vi "GetWaveformData.vi"(5 "Waveform Length (sec)":dbl, 7 "Number of Samples":i32, 8 "error in (no error)":errorcluster, 10 "Waveform":waveform(sgl), 11 "Channel":string) -> (0 "error out":errorcluster, 3 "DataSet":T1)   [LabVIEW 2017, in "EmsaTestPanel.lvlib"]
uses:
  <vilib>/addons/InsightCM/Devices/Shared/Emsa/EmsaTestPanel/EmsaTestPanel.lvlib
  <vilib>/addons/InsightCM/MessageBus/Base/controls/DataSetByteData.ctl
  <vilib>/addons/InsightCM/MessageBus/Base/controls/KeyValuePair.ctl
  <vilib>/addons/InsightCM/Devices/Shared/Cms/CmsTestPanel/CmsTestPanel.lvlib
  <vilib>/addons/InsightCM/Utilities/PropertyHelpers/PropertyHelpers.lvlib
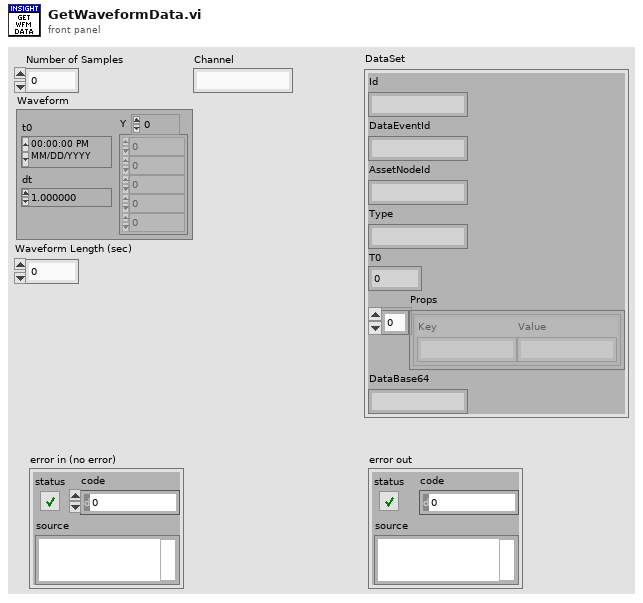
[diagram p1: front panel]
types:
  T1 = typedef "DataSetByteData.ctl" = cluster{"Id":string, "DataEventId":string, "AssetNodeId":string, "Type":string, "T0":i64, "Props":T2[], "DataBase64":string}
  T2 = typedef "KeyValuePair.ctl" = cluster{"Key":string, "Value":string}
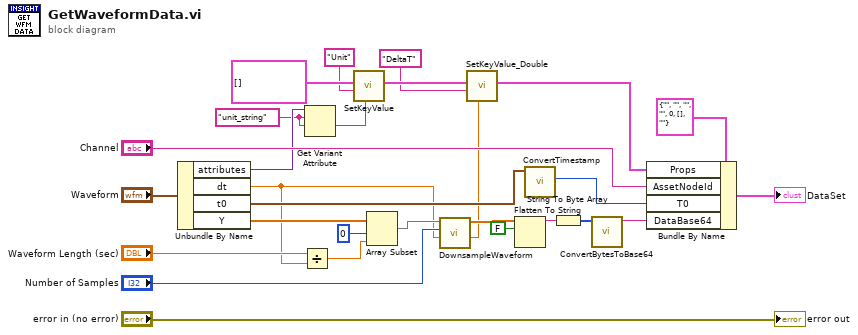
[diagram p0: block diagram]
diagram:
  w22 = "unit_string" ("name")
  n1 = Unbundle By Name("Waveform") -> ("attributes"=w23:variant, "dt"=w1:dbl, "t0"=w9:timestamp, "Y"=w6:sgl[])
  n2 = Divide(x="Waveform Length (sec)", y=w1) -> (x/y=w3:dbl)
  n3 = Get Variant Attribute(Variant=w23, name=w22, default value (empty Variant)=w22) -> (value=w18:string)  [unwired: 1 in, 3 out]
  n4 = call <vilib>:"SetKeyValue.vi"("value"=w18, "key"="Unit", "key value pairs"=T2[] []) -> ("key value pairs out"=w17:T2[])  [unwired: 8 in]
  n5 = Array Subset(array=w6, index=0, length=w3) -> (w5:sgl[])
  n6 = call <vilib>:"DownsampleWaveform.vi"("dt"=w1, "Number of Samples"="Number of Samples", "data"=w5) -> ("new dt"=w2:dbl, "values"=w12:sgl[])  [unwired: 7 in]
  n7 = call <vilib>:"SetKeyValue_Double.vi"("value"=w2, "key"="DeltaT", "key value pairs"=w17) -> ("key value pairs out"=w10:T2[])  [unwired: 8 in]
  n8 = Flatten To String(anything=w12, prepend array or string size? (T)=FALSE) -> (data string=w14:string)  [unwired: 2 in, 2 out]
  n9 = call <vilib>:"ConvertTimestamp.vi"("Time Stamp"=w9) -> ("Timestamp out"=w15:i64)  [unwired: 10 in]
  n10 = String To Byte Array(string=w14) -> (unsigned byte array=w11:u8[])
  n11 = call <vilib>:"ConvertBytesToBase64.vi"("U8 array"=w11) -> ("base64 encoded"=w8:string)  [unwired: 10 in]
  n12 = Bundle By Name(cluster=T1 {"Id"="", "DataEventId"="", "AssetNodeId"="", "Type"="", "T0"=0, "Props"=[], "DataBase64"=""} ("DataSet"), "Props"=w10, "AssetNodeId"="Channel", "T0"=w15, "DataBase64"=w8) -> (→"DataSet":T1)
  "error out" <- "error in (no error)"
